vi "DriveStateController.vi"() -> ()   [LabVIEW 2018]
uses:
  sensors.vi
  dsinstructions.vi
  outputs.vi
panel:
  in  "Deadband":dbl=0.1
  in  "Hysteresis (deg)":dbl=20.0 format="%#_13g"
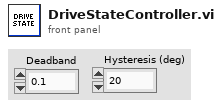
[diagram p1: front panel]
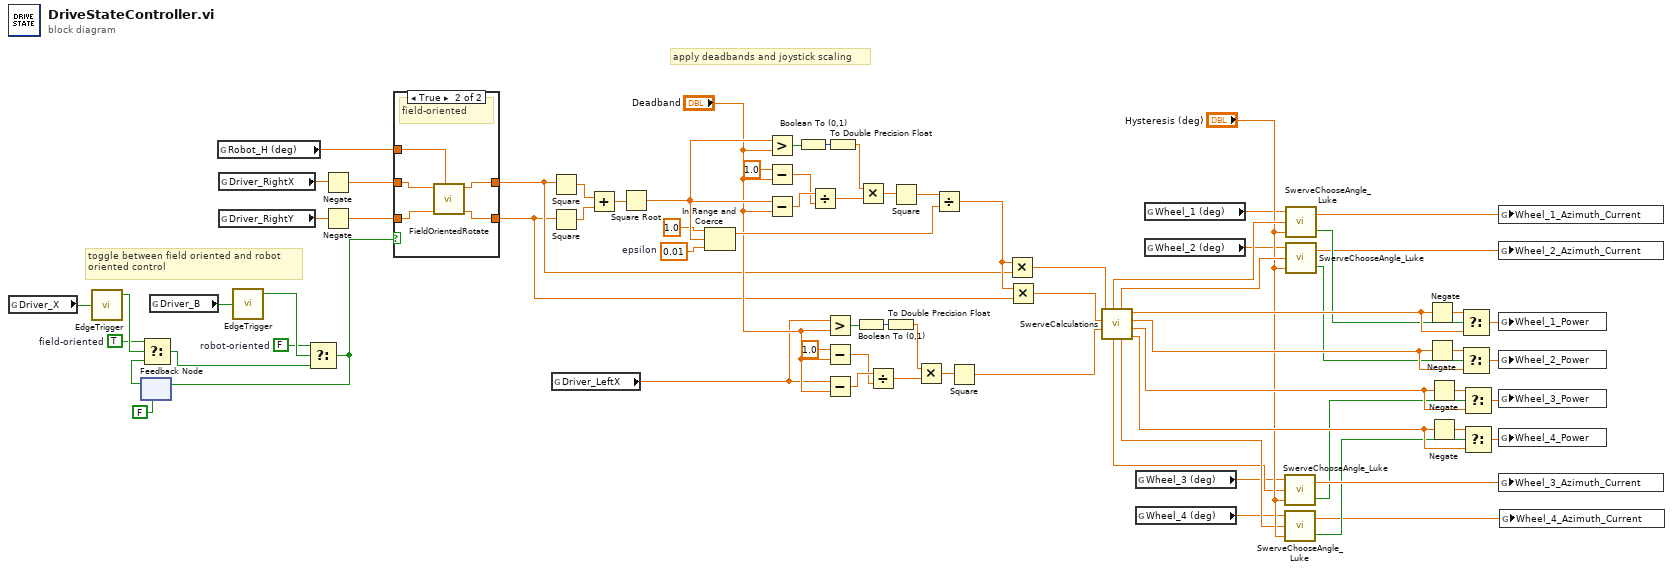
[diagram p0: block diagram]
diagram:
  w5 = TRUE  # field-oriented
  w7 = FALSE  # robot-oriented
  w32 = 0.01  # epsilon
  # "apply deadbands and joystick scaling"
  # "toggle between field oriented and robot \noriented control"
  n1 = global read "dsinstructions.vi" "Driver_X"() -> (w10:bool)
  n2 = call "EdgeTrigger.vi"("Input Signal"=w10) -> ("Rising Edge Trigger"=w6:bool)  [unwired: 2 out]
  n3 = feedback #1(FALSE) -> (w3:bool)
  n4 = Select(t=w5, s=w6, f=w3) -> (s? t:f=w4:bool)
  n5 = global read "dsinstructions.vi" "Driver_B"() -> (w11:bool)
  n6 = global read "sensors.vi" "Robot_H (deg)"() -> (w1:dbl)
  n7 = global read "dsinstructions.vi" "Driver_RightX"() -> (w37:dbl)
  n8 = global read "dsinstructions.vi" "Driver_RightY"() -> (w36:dbl)
  n9 = call "EdgeTrigger.vi"("Input Signal"=w11) -> ("Rising Edge Trigger"=w8:bool)  [unwired: 2 out]
  n10 = Select(t=w7, s=w8, f=w4) -> (s? t:f=w2:bool)
  n11 = feedback-in #1(w2) -> ()
  n12 = Negate(x=w37) -> (-x=w15:dbl)
  n13 = Negate(x=w36) -> (-x=w13:dbl)
  n14 = case shown="True" w2 {
    tunnel: [w78 w83] -> w14
    tunnel: w15 -> [w78 w81]
    tunnel: [w77 w82] -> w12
    tunnel: w13 -> [w77 w80]
    tunnel: w1 -> [_ w79]
    frame False {
      # "robot-oriented"
    }
    frame True {
      # "field-oriented"
      n15 = call "FieldOrientedRotate.vi"("Angle (deg)"=w79, "Y"=w80, "X"=w81) -> ("Y'"=w82:dbl, "X'"=w83:dbl)  [unwired: 7 in]
    }
  }
  n16 = Square(x=w14) -> (x^2=w38:dbl)
  n17 = Square(x=w12) -> (x^2=w39:dbl)
  n18 = global read "dsinstructions.vi" "Driver_LeftX"() -> (w17:dbl)
  n19 = Add(x=w38, y=w39) -> (x+y=w35:dbl)
  n20 = Square Root(x=w35) -> (sqrt(x)=w31:dbl)
  n21 = In Range and Coerce(upper limit=1.0, x=w31, lower limit=w32) -> (coerced(x)=w33:dbl)  [unwired: 1 out]
  n22 = Greater?(x=w31, y="Deadband") -> (0:w47:bool)
  n23 = Subtract(x=1.0, y="Deadband") -> (x-y=w41:dbl)
  n24 = Subtract(x=w31, y="Deadband") -> (x-y=w43:dbl)
  n25 = Boolean To (0,1)(Boolean=w47) -> (0, 1=w46:i16)
  n26 = Divide(x=w43, y=w41) -> (x/y=w40:dbl)
  n27 = Greater?(x=w17, y="Deadband") -> (0:w26:bool)
  n28 = Subtract(x=1.0, y="Deadband") -> (x-y=w20:dbl)
  n29 = Subtract(x=w17, y="Deadband") -> (x-y=w22:dbl)
  n30 = To Double Precision Float(number=w46) -> (double precision float=w45:dbl)
  n31 = Boolean To (0,1)(Boolean=w26) -> (0, 1=w25:i16)
  n32 = Multiply(x=w45, y=w40) -> (x*y=w44:dbl)
  n33 = Divide(x=w22, y=w20) -> (x/y=w19:dbl)
  n34 = To Double Precision Float(number=w25) -> (double precision float=w24:dbl)
  n35 = Square(x=w44) -> (x^2=w34:dbl)
  n36 = Multiply(x=w24, y=w19) -> (x*y=w23:dbl)
  n37 = Divide(x=w34, y=w33) -> (x/y=w29:dbl)
  n38 = Square(x=w23) -> (x^2=w16:dbl)
  n39 = Multiply(x=w29, y=w14) -> (x*y=w28:dbl)
  n40 = Multiply(x=w29, y=w12) -> (x*y=w27:dbl)
  n41 = call "SwerveCalculations.vi"("j2x"=w16, "j1y"=w27, "j1x"=w28) -> ("magnitude4"=w74:dbl, "magnitude3"=w73:dbl, "magnitude2"=w71:dbl, "magnitude1"=w72:dbl, "Wheel Angle4"=w67:dbl, "Wheel Angle2"=w69:dbl, "Wheel Angle3"=w63:dbl, "wheel angle 1"=w70:dbl)  [unwired: 1 in]
  n42 = global read "sensors.vi" "Wheel_3 (deg)"() -> (w62:dbl)
  n43 = global read "sensors.vi" "Wheel_4 (deg)"() -> (w48:dbl)
  n44 = global read "sensors.vi" "Wheel_1 (deg)"() -> (w50:dbl)
  n45 = global read "sensors.vi" "Wheel_2 (deg)"() -> (w49:dbl)
  n46 = call "SwerveChooseAngle_Luke.vi"("Hysteresis (deg)"="Hysteresis (deg)", "Goal Angle (deg)"=w63, "Current Angle (deg)"=w62) -> ("Invert Speed  Motor (?)"=w65:bool, "Angular Distance (deg)"=w66:dbl)
  n47 = call "SwerveChooseAngle_Luke.vi"("Hysteresis (deg)"="Hysteresis (deg)", "Goal Angle (deg)"=w67, "Current Angle (deg)"=w48) -> ("Invert Speed  Motor (?)"=w64:bool, "Angular Distance (deg)"=w53:dbl)
  n48 = call "SwerveChooseAngle_Luke.vi"("Hysteresis (deg)"="Hysteresis (deg)", "Goal Angle (deg)"=w70, "Current Angle (deg)"=w50) -> ("Invert Speed  Motor (?)"=w57:bool, "Angular Distance (deg)"=w55:dbl)
  n49 = call "SwerveChooseAngle_Luke.vi"("Hysteresis (deg)"="Hysteresis (deg)", "Goal Angle (deg)"=w69, "Current Angle (deg)"=w49) -> ("Invert Speed  Motor (?)"=w56:bool, "Angular Distance (deg)"=w54:dbl)
  n50 = Negate(x=w72) -> (-x=w61:dbl)
  n51 = Negate(x=w71) -> (-x=w59:dbl)
  n52 = Negate(x=w73) -> (-x=w76:dbl)
  n53 = Negate(x=w74) -> (-x=w52:dbl)
  n54 = Select(t=w61, s=w57, f=w72) -> (s? t:f=w60:dbl)
  n55 = Select(t=w59, s=w56, f=w71) -> (s? t:f=w58:dbl)
  n56 = Select(t=w76, s=w65, f=w73) -> (s? t:f=w75:dbl)
  n57 = Select(t=w52, s=w64, f=w74) -> (s? t:f=w51:dbl)
  n58 = global write "outputs.vi" "Wheel_1_Azimuth_Current"(w55) -> ()
  n59 = global write "outputs.vi" "Wheel_2_Azimuth_Current"(w54) -> ()
  n60 = global write "outputs.vi" "Wheel_1_Power"(w60) -> ()
  n61 = global write "outputs.vi" "Wheel_2_Power"(w58) -> ()
  n62 = global write "outputs.vi" "Wheel_3_Power"(w75) -> ()
  n63 = global write "outputs.vi" "Wheel_4_Power"(w51) -> ()
  n64 = global write "outputs.vi" "Wheel_3_Azimuth_Current"(w66) -> ()
  n65 = global write "outputs.vi" "Wheel_4_Azimuth_Current"(w53) -> ()
